vi "Main_SubVI_CRC.vi"(8 "Error In":errorcluster, 11 "Command":string) -> (0 "Error Out":errorcluster, 2 "CRC Result":string, 3 "CRC":u32)   [LabVIEW 2015]
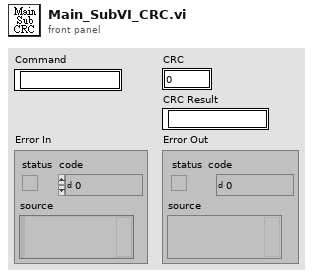
[diagram p1: front panel]
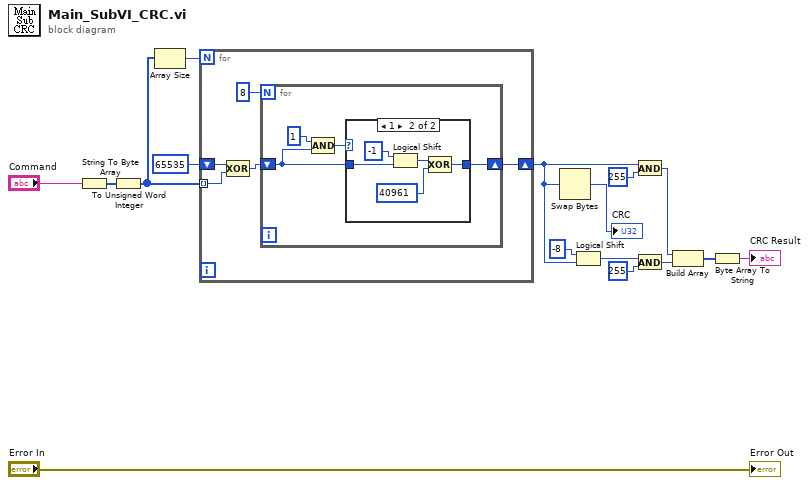
[diagram p0: block diagram]
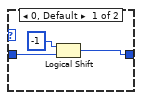
[diagram p2: hidden frame]
diagram:
  n1 = String To Byte Array(string="Command") -> (unsigned byte array=w15:u8[])
  n2 = To Unsigned Word Integer(number=w15) -> (unsigned 16bit integer=w3:u16[])
  n3 = Array Size(array=w3) -> (size(s)=w2:i32)
  n4 = for {
    N: w2 -> [_]
    shift-right: [w19] -> w10
    shift-left: u16 65535 -> [w20]
    tunnel: w3 -> [w18] mode=indexing
    n5 = Compound Arithmetic op=XOR(w20, w18) -> (w21:u32)
    n6 = for {
      N: 8 -> [_]
      shift-right: [w24] -> w19
      shift-left: w21 -> [w23]
      n7 = Compound Arithmetic op=AND(u16 1, w23) -> (w22:u32)
      n8 = case shown="1" w22 {
        tunnel: [w27 w32] -> w24
        tunnel: w23 -> [w26 w29]
        frame 0, Default {
          n9 = Logical Shift(y=i16 -1, x=w26) -> (x << y=w27:u32)
        }
        frame 1 {
          n10 = Logical Shift(y=i16 -1, x=w29) -> (x << y=w31:u32)
          n11 = Compound Arithmetic op=XOR(w31, u32 40961) -> (w32:u32)
        }
      }
    }
  }
  n12 = Swap Bytes(anything=w10) -> (byte swapped=→"CRC":u32)
  n13 = Logical Shift(y=i16 -8, x=w10) -> (x << y=w12:u32)
  n14 = And(x=w10, y=u16 255) -> (x .and. y?=w9:u32)
  n15 = And(x=w12, y=u16 255) -> (x .and. y?=w8:u32)
  n16 = Build Array(w9, w8) -> (w7:u32[])
  n17 = Byte Array To String(unsigned byte array=w7) -> (string=→"CRC Result":string)
  "Error Out" <- "Error In"
